vi "Log instrument initialization.vi"(8 "error in (no error)":errorcluster, 10 "Instruments with errors":refnum<class "nLight Instrument.lvclass">[](array[class]), 11 "Initialized instruments":refnum<class "nLight Instrument.lvclass">[](array[class])) -> (0 "error out":errorcluster)   [LabVIEW 2018]
doc: "Creates brief and verbose entries for the instrument initialization. This VI is intended to be placed immediately following any instance of the \"Start station instruments\" VI from the station configuration class."
uses:
  <instrlib>/nLight Instruments/nLight Instrument/nLight Instrument.lvclass
  <userlib>/nLight Tidbits/Logging/Controls/Logging type choice.ctl
  <vilib>/Utility/error.llb/Clear Errors.vi
  <userlib>/nLight Error Handling/Log any errors.vi
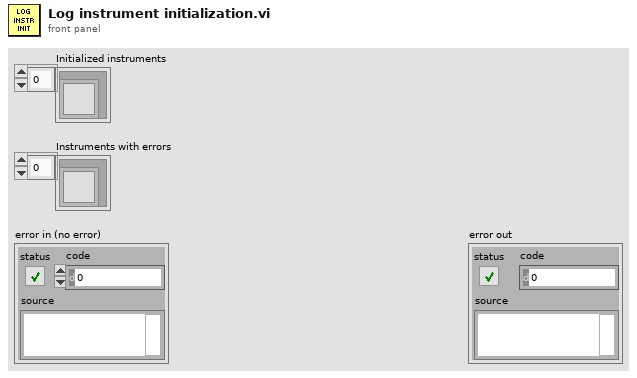
[diagram p1: front panel]
types:
  T1 = typedef "Logging type choice.ctl" = enum16{"No log type selected", "Testing start/stop", "Test progress", "Station startup/shutdown", "Station config change", "Recipe load/change", "Inventory transaction", "Instrument", "Debug"}
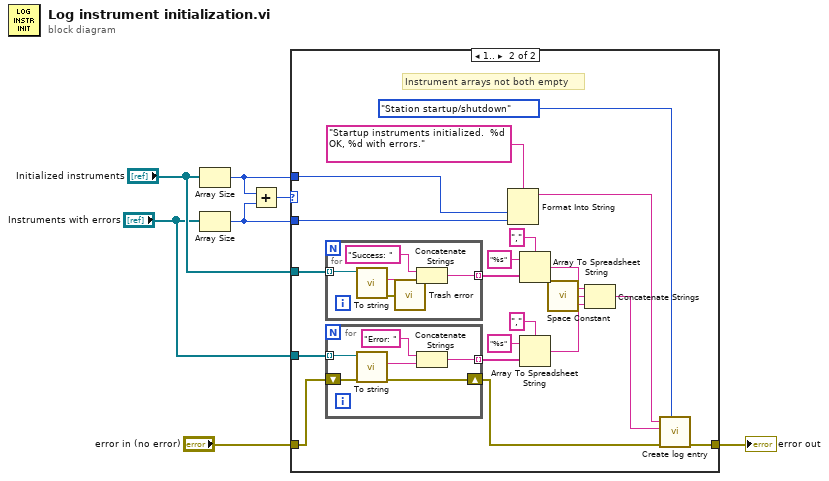
[diagram p0: block diagram]
diagram:
  n1 = Array Size(array="Initialized instruments") -> (size(s)=w2:i32)
  n2 = Array Size(array="Instruments with errors") -> (size(s)=w3:i32)
  n3 = Add(x=w2, y=w3) -> (x+y=w4:i32)
  n4 = case shown="1.." w4 {
    tunnel: "error in (no error)" -> [w8 w10]
    tunnel: [w8 w28] -> w7
    tunnel: w3 -> [_ w25]
    tunnel: w2 -> [_ w26]
    tunnel: "Initialized instruments" -> [_ w22]
    tunnel: "Instruments with errors" -> [_ w15]
    frame ..0 {
      # "Instrument arrays both empty"
    }
    frame 1.. {
      # "Instrument arrays not both empty"
      n5 = for {
        tunnel: w22 -> [w38] mode=indexing
        tunnel: [w36] -> w21 mode=indexing
        n6 = call-dynamic "To string.vi"("nLight Instrument in"=w38) -> ("error out"=w35:errorcluster, "String"=w37:string)  [unwired: 8 in, 1 out]
        n7 = call <userlib>:"Trash error.vi"("error in"=w35) -> ()  [unwired: 15 in]
        n8 = Concatenate Strings("Success: " ("string"), w37) -> (w36:string)
      }
      n9 = for {
        tunnel: w15 -> [w33] mode=indexing
        tunnel: [w31] -> w16 mode=indexing
        shift-right: [w29] -> w9
        shift-left: w10 -> [w30]
        n10 = call-dynamic "To string.vi"("error in (no error)"=w30, "nLight Instrument in"=w33) -> ("error out"=w29:errorcluster, "String"=w32:string)  [unwired: 7 in, 1 out]
        n11 = Concatenate Strings("Error: " ("string"), w32) -> (w31:string)
      }
      n12 = Format Into String(format string="Startup instruments initialized.  %d OK, %d with errors." ("Brief log entry"), w26, w25) -> (resulting string=w24:string)  [unwired: 2 in, 1 out]
      n13 = Array To Spreadsheet String(delimiter (Tab)=",", array=w21, 3:"%s" ("format string")) -> (spreadsheet string=w14:string)
      n14 = Array To Spreadsheet String(delimiter (Tab)=",", array=w16, 3:"%s" ("format string")) -> (spreadsheet string=w12:string)
      n15 = call <vilib>:"Space Constant.vi"() -> ("String"=w13:string)
      n16 = Concatenate Strings(w14, w13, w12) -> (w11:string)
      n17 = call <userlib>:"Create log entry.vi"("Logging type choice"=Logging_type_choice."Station startup/shutdown", "error in (no error)"=w9, "Verbose log addition (none)"=w11, "Brief log entry"=w24) -> ("error out"=w28:errorcluster)  [unwired: 7 in]
    }
  }
  "error out" <- w7
